vi "Amplifiers.vi"() -> ()   [LabVIEW 2019]
doc: "The NI ELVIS III Custom FPGA Project template acquires button data from the onboard button and displays the button value on a Boolean indicator."
uses:
  <vilib>/Platform/TimedLoop/XDataNode/timing_clust.ctl
  <vilib>/Platform/TimedLoop/XDataNode/nitl_modes.ctl
  <vilib>/Platform/TimedLoop/XDataNode/wakeup.ctl
  <vilib>/Platform/TimedLoop/XDataNode/XDataNode.xnode
  <vilib>/Platform/TimedLoop/XDataNode/XDNodeRunTimeDep.lvlib
panel:
  in  "PWM Reverse":bool
  in  "Linear Amplifier\nCommand Gain":sgl
  in  "Amplifier":u16(ring) items=["Linear", "PWM"]
  out "Load Current \n(mA)":sgl
  out "Load Current":sgl(graph)=0.7266998
  out "Error Out":errorcluster
  out "DC Motor \nSpeed (RPM)":dbl=0.023283064370807974 format="%#.0f"
  out "DC Motor Speed":dbl(graph)=0.023283064370807974
  in  "Amplifier Command":sgl(knob) min=-5 max=5 step=0.01 scale=-1.0..1.0
  in  "Stop Button":bool
  # "Mechatronic Actuators Board"
  # "Amplifiers"
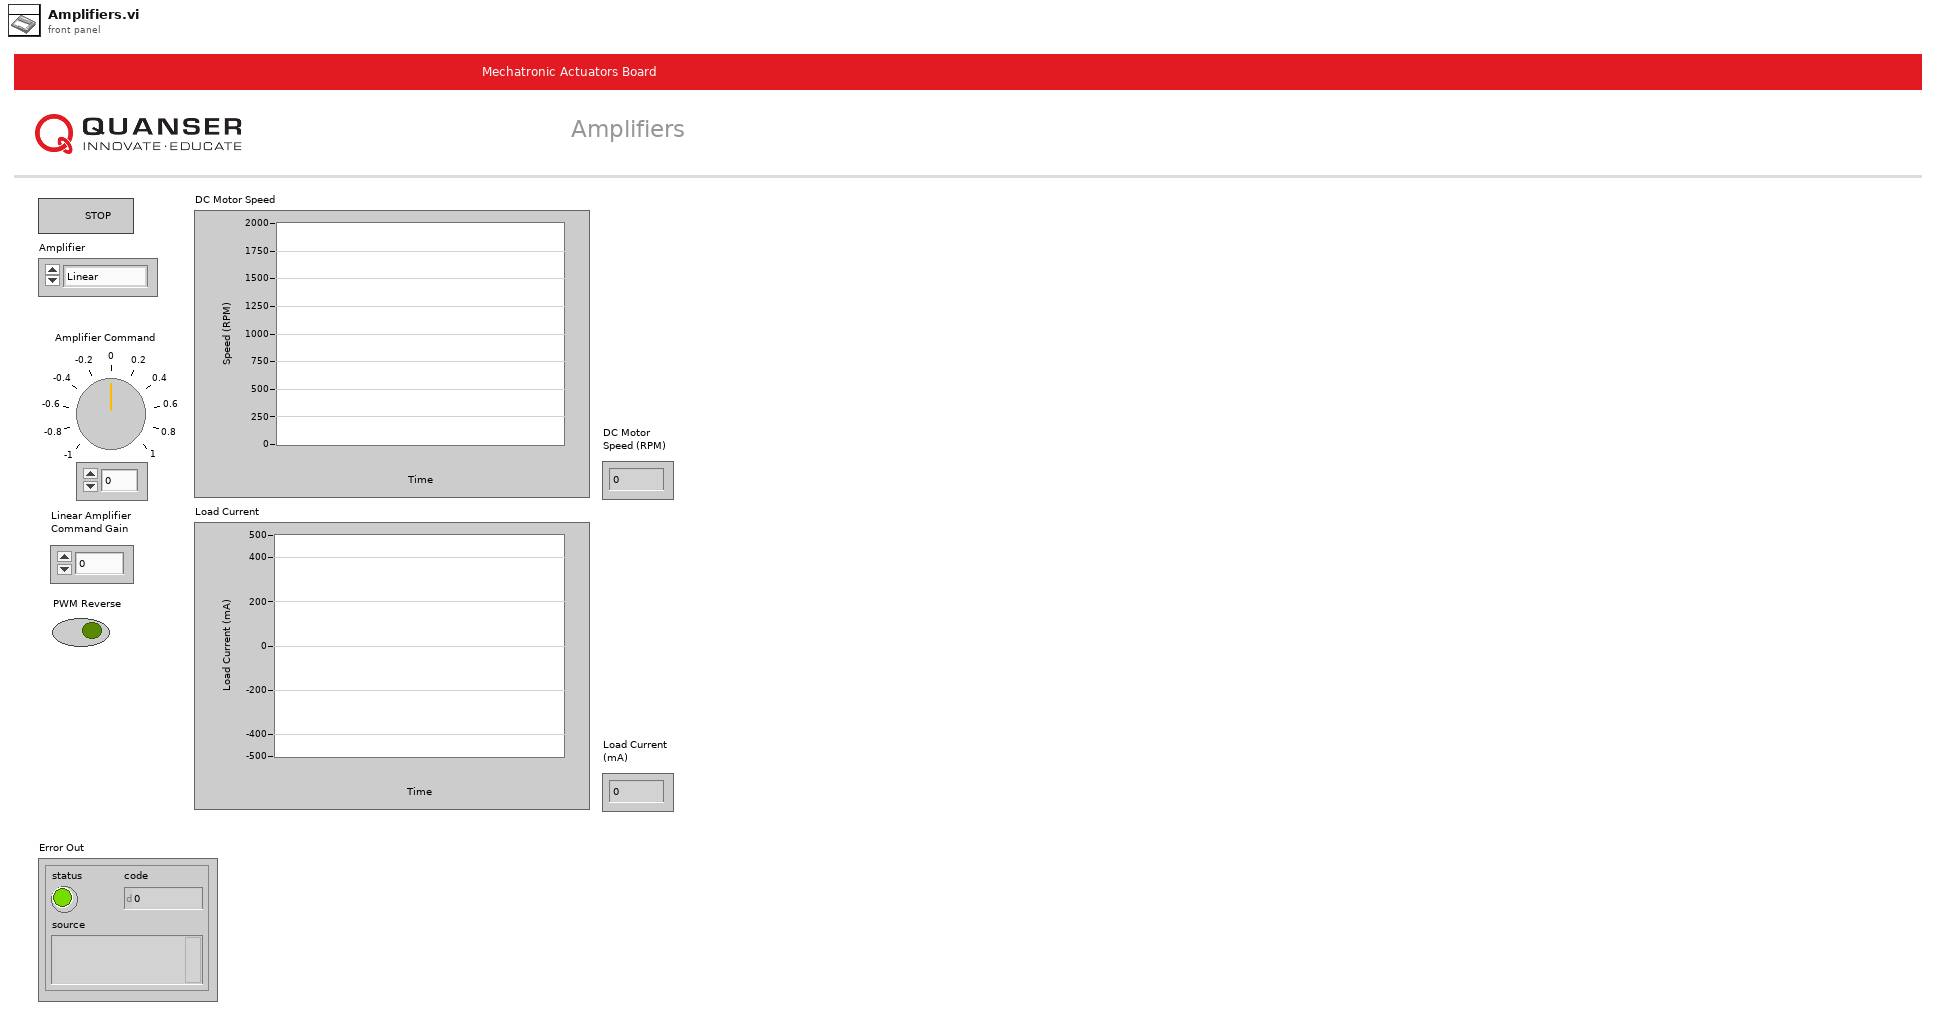
[diagram p1: front panel]
types:
  T1 = typedef "XDNodeRunTimeDep.lvlib/timing_clust.ctl" = cluster{"Expected End [f-1]":u64, "Actual End [f-1]":u64, "Finished Late? [f-1]":bool, "Expected End [i-1]":u64, "Actual End [i-1]":u64, "Finished Late? [i-1]":bool, "Expected Start [i]":u64, "Actual Start [i]":u64, "Expected Start [f]":u64, "Actual Start [f]":u64, "Source Name":string, "Structure Name":string, "Period":i64, "Deadline":i64, "Offset":i64, "Start":i64, "Priority":i32, "Timeout":i32, "Mode":T2, "Wakeup Reason":T3, "Error":errorcluster, "Source Type":string, "Secondary Source Type":string, "Global End Time":u64, "Global Start Time":u64, "Frame Duration":u64, "Iteration Duration":u64, "Assigned CPU":i32, "I/O Scan Engine Mode":u32}
  T2 = typedef "XDNodeRunTimeDep.lvlib/nitl_modes.ctl" = enum32{"No Change", "Process missed periods, maintain original phase", "Discard missed periods, maintain original phase", "Process missed periods, ignore original phase", "Discard missed periods, ignore original phase"}
  T3 = typedef "XDNodeRunTimeDep.lvlib/wakeup.ctl" = enum32{"Normal", "Aborted", "Asynchronous wakeup", "Timing source error", "Timed loop error", "Timeout"}
  T4 = typedef "Actuators IO Cluster.ctl" = cluster{"Error":errorcluster, "FPGA Ref":refnum<k20>}
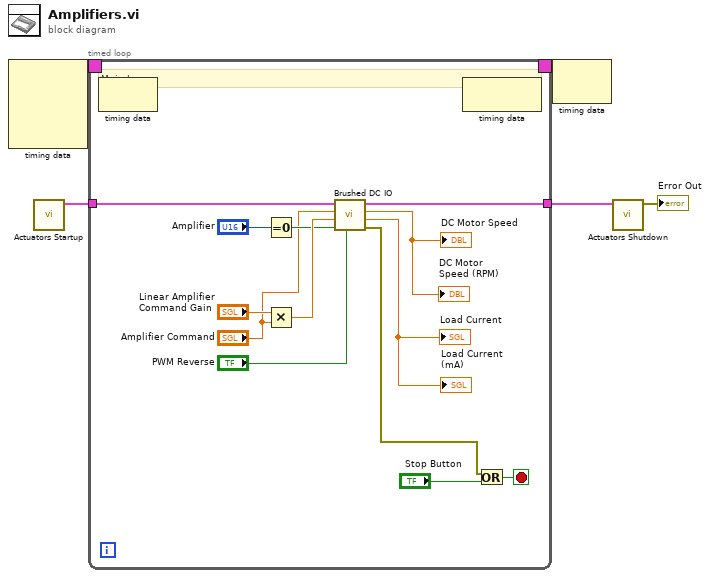
[diagram p0: block diagram]
diagram:
  n1 = node-c288() -> (w5:T1)  [unwired: 4 in]
  n2 = call "Actuators Startup.vi"() -> ("IO Cluster OUT"=w3:T4)  [unwired: 11 in]
  n3 = timed-loop {
    timing: w5 -> [_]
    timing-out: [_] -> w4
    tunnel: w3 -> [w16]
    tunnel: [w15] -> w2
    stop <- w18 stop-if-true
    # "Main Loop"
    n4 = node-c288() -> ()  [unwired: 1 in, 1 out]
    n5 = Equal To 0?(x="Amplifier") -> (x = 0?=w9:bool)
    n6 = Multiply(x="Linear Amplifier\nCommand Gain", y="Amplifier Command") -> (x*y=w13:sgl)
    n7 = call "Brushed DC IO.vi"("Brushed DC PWM Reverse"="PWM Reverse", "Linear Amplifier Enable"=w9, "Brushed DC Motor Linear"=w13, "Brushed DC Motor PWM"="Amplifier Command", "IO Cluster IN"=w16) -> ("Error Out"=w14:errorcluster, "Brushed DC Motor Filtered Current"=→"Load Current \n(mA)" →"Load Current":sgl, "Brushed DC Motor Speed (RPM)"=→"DC Motor Speed" →"DC Motor \nSpeed (RPM)":dbl, "IO Cluster OUT"=w15:T4)  [unwired: 3 in]
    n8 = node-c288() -> ()  [unwired: 1 in, 1 out]
    n9 = Or(x=w14, y="Stop Button") -> (x .or. y?=w18:bool)
  }
  n10 = node-c288(w4) -> ()  [unwired: 1 out]
  n11 = call "Actuators Shutdown.vi"("IO Cluster IN"=w2) -> ("Error Out"=→"Error Out":errorcluster)  [unwired: 10 in]
